vi "Handle Value Change.vi"(5 "VolatusAPI":refnum<class "VolatusAPI.lvclass">, 7 "CtlRef":refnum<vi>, 8 "error in (no error)":errorcluster, 9 "NewVal":variant, 10 "OldVal":variant, 11 "HtmlButtonControl in":refnum<class "HttpButtonControl.lvclass">) -> (0 "error out":errorcluster, 3 "HtmlButtonControl out":refnum<class "HttpButtonControl.lvclass">)   [LabVIEW 2020, in "VolatusGUIElements.lvlib" / "HttpButtonControl.lvclass"]
uses:
  HttpButtonControl.lvclass
  HttpButtonControl.lvclass/HttpButtonControl.ctl
  Volatus/VolatusAPI/VolatusAPI.lvclass
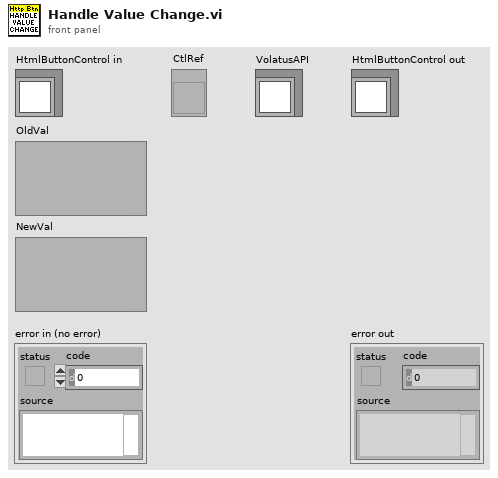
[diagram p1: front panel]
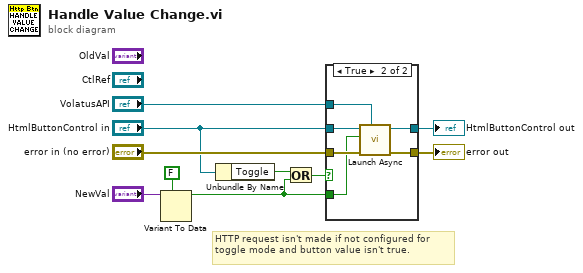
[diagram p0: block diagram]
diagram:
  # "HTTP request isn't made if not configured for toggle mode and button value isn't true."
  n1 = Variant To Data(type=FALSE, Variant="NewVal") -> (data=w2:bool)  [unwired: 1 in, 1 out]
  n2 = Unbundle By Name("HtmlButtonControl in") -> ("Toggle"=w3:bool)
  n3 = Or(x=w3, y=w2) -> (x .or. y?=w1:bool)
  n4 = case shown="True" w1 {
    tunnel: "error in (no error)" -> [w11 w18]
    tunnel: [w11 w17] -> w7
    tunnel: [w12 w16] -> w6
    tunnel: "VolatusAPI" -> [_ w15]
    tunnel: "HtmlButtonControl in" -> [w12 w14]
    tunnel: w2 -> [_ w13]
    frame False {
    }
    frame True {
      n5 = call "Launch Async.vi"("VolatusAPI"=w15, "error in (no error)"=w18, "Value"=w13, "HtmlButtonControl in"=w14) -> ("error out"=w17:errorcluster, "HtmlButtonControl out"=w16:refnum<class "HttpButtonControl.lvclass">)  [unwired: 6 in]
    }
  }
  "error out" <- w7
  "HtmlButtonControl out" <- w6
